vi "Add Test Case.vi"(8 "Error In (No Error)":errorcluster, 9 "Test Case Atrributes":T1={"name"="", "assertions"=-1, "time"=-1.0, "timestamp"=-1.0, "classname"="", "status"="", "class"="", "file"="", "line"="", "log"="", "group"="", "url"=""}, 10 "Testsuite Ref In":refnum<k20>, 11 "File Ref In":refnum<k20>) -> (0 "error out":errorcluster, 2 "Testcase Ref":refnum<k20>, 3 "File Ref Out":refnum<k20>, 5 "Testsuite Ref Out":refnum<k20>)   [LabVIEW 2013, in "JUnit API.lvlib"]
uses:
  JUnit API.lvlib
  Controls/Test Case Attributes.ctl
  <vilib>/NI/Simple XML/_polymorphics/Create Tag - Child.vi
  <vilib>/NI/Simple XML/Simple XML.lvlib
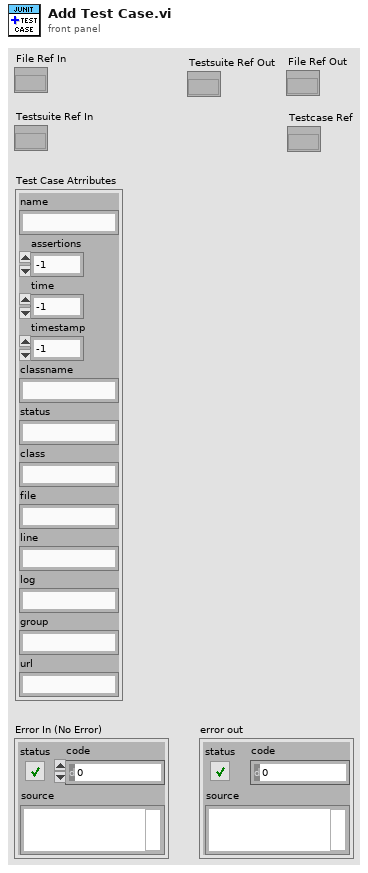
[diagram p1: front panel]
types:
  T1 = typedef "JUnit API.lvlib/Test Case Attributes.ctl" = cluster{"name":string, "assertions":i32, "time":dbl, "timestamp":dbl, "classname":string, "status":string, "class":string, "file":string, "line":string, "log":string, "group":string, "url":string}
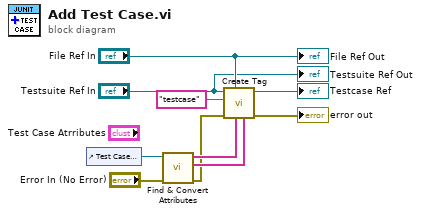
[diagram p0: block diagram]
diagram:
  n1 = control-ref of="Test Case Atrributes"() -> (w1:refnum<vi>)
  n2 = call "Find & Convert Attributes.vi"("Error In"="Error In (No Error)", "Cluster in"=w1) -> ("Error Out"=w2:errorcluster, "Attribute Values"=w4:string[], "Attribute Names"=w5:string[])  [unwired: 7 in]
  n3 = call-poly <vilib>:"Create Tag.vi"("Attr Values"=w4, "Attr Names"=w5, "DOM Document reference"="File Ref In", "error in (no error)"=w2, "Tag Name"="testcase", "Parent Element reference"="Testsuite Ref In") -> ("error out"=→"error out":errorcluster, "Child Element reference"=→"Testcase Ref":refnum<k20>)  [unwired: 4 in]
  "File Ref Out" <- "File Ref In"
  "Testsuite Ref Out" <- "Testsuite Ref In"
